vi "readPLCConfigFile.vi"(8 "Error In":errorcluster, 11 "PLC Config File Path":path) -> (0 "Error Out":errorcluster, 1 "Numeric":u16, 2 "Port":i32, 3 "IP Address":string)   [LabVIEW 2018]
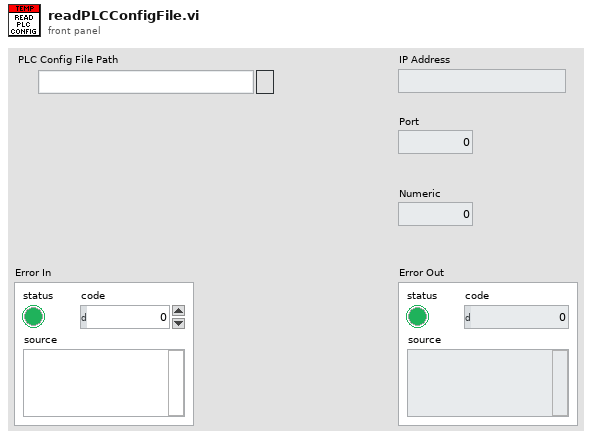
[diagram p1: front panel]
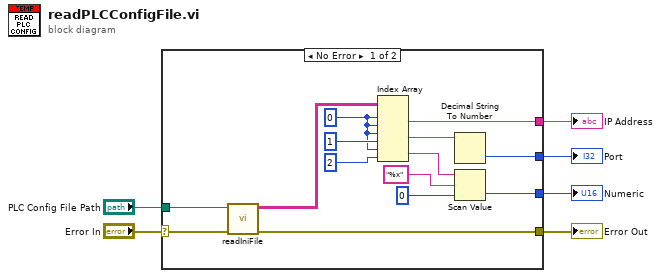
[diagram p0: block diagram]
diagram:
  n1 = case shown="No Error" "Error In" {
    selector: "Error In" -> [w20 w21]
    tunnel: [w19 w21] -> w4
    tunnel: "PLC Config File Path" -> [w18 _]
    tunnel: [w16 _] -> w3
    tunnel: [w12 _] -> w2
    tunnel: [w8 _] -> w1
    frame No Error {
      w14 = 0 ("index (row)")
      n2 = call "readIniFile.vi"("Error In"=w20, "File Path Control"=w18) -> ("Error Out"=w19:errorcluster, "Value"=w17:string[][])  [unwired: 8 in]
      n3 = Index Array(array=w17, index (row) #1=w14, index (col) #1=w14, index (row) #2=w14, index (col) #2=1 ("index (row)"), index (row) #3=w14, index (col) #3=2 ("disabled index (col)")) -> (element #1=w16:string, element #2=w10:string, element #3=w9:string)
      n4 = Decimal String To Number(string=w10) -> (number=w12:i32)  [unwired: 2 in, 1 out]
      n5 = Scan Value(string=w9, format string="%x", default (0 dbl)=u16 0) -> (value=w8:u16)  [unwired: 1 out]
    }
    frame Error {
    }
  }
  "IP Address" <- w3
  "Error Out" <- w4
  "Port" <- w2
  "Numeric" <- w1
